vi "Core.vi"(8 "error in (no error)":errorcluster, 11 "Test 1 in":refnum<class "Test Caller.lvclass">) -> (0 "error out":errorcluster, 3 "Actor out":refnum<class "Actor.lvclass">)   [LabVIEW 2020, in "Scratchpad.lvlib" / "Test Caller.lvlib" / "Test Caller.lvclass"]
uses:
  Test Caller.lvclass
  C:/dev/lv20CE/relink/lv-artifex/Artifex/Actor/Actor.lvclass
  Artifex/Actor/Actor.lvclass
  Test Caller.lvclass/Test Caller.ctl
  Artifex/Actor Proxy/Actor API.lvclass/Actor API.ctl
  Artifex/Actor Proxy/Send Message.vi
  Test 1/Test 1/Test 1.lvclass
  Test 1/Test 1 API/Test 1 API.lvclass
  C:/dev/lv20CE/relink/lv-artifex/Artifex/Actor Proxy/Actor API.lvclass
  Test Caller API/Test Caller API.lvclass
  Artifex/Stop Msg/Stop Msg.lvclass
  C:/dev/lv20CE/relink/lv-artifex/Artifex/Message/Message.lvclass
  Artifex/Actor/Launch Nested.vi
  Artifex/Priority Message Queue/Priority Enqueue.vi
  Artifex/Actor Proxy/Actor API.lvclass
  <vilib>/ptbypt/NI_PtbyPt.lvlib
panel:
  in  "Start":bool
  out "Count":i32
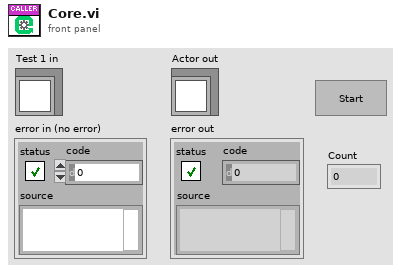
[diagram p1: front panel]
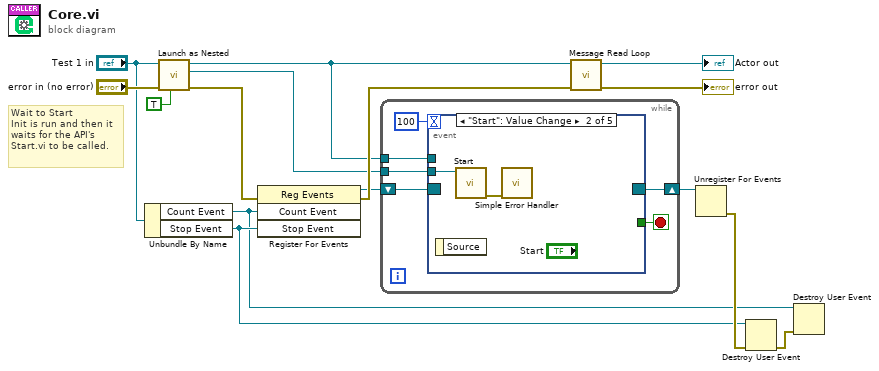
[diagram p0: block diagram]
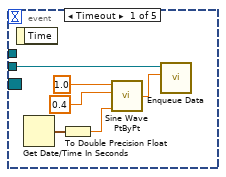
[diagram p2: hidden frame]
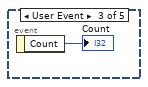
[diagram p3: hidden frame]
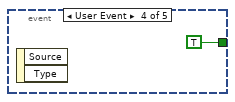
[diagram p4: hidden frame]
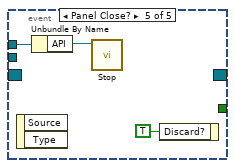
[diagram p5: hidden frame]
diagram:
  # "Wait to Start\nInit is run and then it waits for the API's Start.vi to be called."
  n1 = Unbundle By Name("Test 1 in") -> ("Count Event"=w6:refnum<user-event>, "Stop Event"=w7:refnum<user-event>)
  n2 = call "Launch as Nested.vi"("Wait to Start (F)"=TRUE, "error in (no error)"="error in (no error)", "Caller In"="Test 1 in") -> ("error out"=w3:errorcluster, "Test 1 API"=w2:refnum<class "Test 1 API.lvclass">, "Caller"=w4:refnum<class "Test Caller.lvclass">)  [unwired: 6 in]
  n3 = register-events(error in=w3, w6, w7) -> (reference out=w11:refnum<event-registration>, error out=w12:errorcluster)  [unwired: 1 in]
  n4 = while {
    shift-right: [w19] -> w10
    shift-left: w11 -> [w20]
    tunnel: w4 -> [w17]
    tunnel: w2 -> [w16]
    stop <- w18 stop-if-true
    n5 = event shown="[1] \"Start\": Value Change" {
      selector: w20 -> [_ _ _ _ _]
      dyn-events: [_ _ _ _ _] -> w19
      timeout: 100 -> [_ _ _ _ _]
      tunnel: [_ _ _ TRUE _] -> w18
      tunnel: w17 -> [_ _ _ _ w33]
      tunnel: w16 -> [w27 w29 _ _ _]
      event Timeout {
        n6 = event-data() -> ()  [unwired: 1 in, 1 out]
        n7 = Get Date/Time In Seconds() -> (seconds since 1Jan1904=w23:timestamp)
        n8 = To Double Precision Float(number=w23) -> (double precision float=w22:dbl)
        n9 = call <vilib>:"Sine Wave PtByPt.vi"("time"=w22, "frequency"=0.4, "amplitude"=1.0) -> ("sine wave"=w24:dbl)  [unwired: 1 in]
        n10 = call "Enqueue Data.vi"("Data"=w24, "Test 1 API in"=w27) -> ()  [unwired: 8 in, 2 out]
      }
      event "Start": Value Change {
        n11 = event-data() -> ()  [unwired: 1 in, 1 out]
        n12 = call "Start.vi"("Actor API in"=w29) -> ("error out"=w28:errorcluster)  [unwired: 9 in, 1 out]
        n13 = call <vilib>:"Simple Error Handler.vi"("error in (no error)"=w28) -> ()  [unwired: 4 in, 5 out]
      }
      event User Event {
        n14 = event-data() -> ("Count"=→"Count":i32)  [unwired: 1 in]
      }
      event User Event {
        n15 = event-data() -> ()  [unwired: 1 in, 2 out]
      }
      event Panel Close? {
        n16 = event-data() -> ()  [unwired: 1 in, 2 out]
        n17 = Unbundle By Name(w33) -> ("API"=w32:refnum<class "Test Caller API.lvclass">)
        n18 = call "Stop.vi"("Actor API in"=w32) -> ()  [unwired: 9 in, 2 out]
        n19 = event-data("Discard?"=TRUE) -> ()  [unwired: 1 in, 1 out]
      }
    }
  }
  n20 = call "Message Read Loop.vi"("error in (no error)"=w12, "Actor in"=w4) -> ("error out"=→"error out":errorcluster, "Actor out"=→"Actor out":refnum<class "Actor.lvclass">)  [unwired: 8 in]
  n21 = Unregister For Events(event registration refnum=w10) -> (error out=w9:errorcluster)  [unwired: 1 in]
  n22 = Destroy User Event(user event=w7, error in=w9) -> (error out=w8:errorcluster)
  n23 = Destroy User Event(user event=w6, error in=w8) -> ()  [unwired: 1 out]
